vi "J1939 - Tool.vi"() -> ()   [LabVIEW 2019, in "J1939 Workspace Tool.lvlib"]
uses:
  J1939 Workspace Tool.lvlib
  NationalInstruments.VeriStand.SystemStorage
  SubModules/CAN-Streaming-Support/Source/Addon/Addon Shared/Types/Type Filter.ctl
  SubModules/CAN-Streaming-Support/Source/Addon/Addon Shared/Types/Direction Filter.ctl
  Workspace Shared/Types/UI.StateVariables.ctl
  <vilib>/NI VeriStand/Display Template Support/DisplayTemplateSupport.llb/enum_Display Template Handler Minimal To Widget Msg.ctl
  <vilib>/NI VeriStand/Execution/Workspace/SystemStateRegEventRef.ctl
  <vilib>/NI VeriStand/Execution/Workspace/Target State Info.ctl
  <vilib>/NI VeriStand/Execution/Workspace/Target State.ctl
  Workspace Shared/Types/Private Data.ctl
  <vilib>/NI/STM/TCP/TCP Connection Info.ctl
  <vilib>/NI/STM/SubVIs/MetaDataElement.ctl
  Addon/Addon Shared/Types/Error Cluster.ctl
  Addon/Addon Shared/Types/Error Types.ctl
  <vilib>/NI VeriStand/Display Template Support/DisplayTemplateSupport.llb/enum_Display Template Handler Minimal To Workspace.ctl
  <vilib>/NI VeriStand/Execution/Workspace/WorkspaceAPI.ctl
  <vilib>/NI VeriStand/Execution/Workspace/SystemStateEventRef.ctl
  Workspace Shared/Types/UI.Refs.ctl
  SubModules/CAN-Streaming-Support/Source/UIs/Workspace Shared/Types/Host Stream Queue Refs.ctl
  SubModules/CAN-Streaming-Support/Source/UIs/Workspace Shared/Types/Host Stream Queue Type.ctl
  SubModules/CAN-Streaming-Support/Source/UIs/Workspace Shared/Types/Host Stream Queue Command.ctl
  <vilib>/xnet/xnet.llb/XNET Frame CAN.ctl
  <vilib>/xnet/xnet.llb/XNET Frame Type CAN.ctl
  SubModules/CAN-Streaming-Support/Source/UIs/Workspace Shared/Types/Host Stream Engine Parameters.ctl
  SubModules/CAN-Streaming-Support/Source/Addon/Addon Shared/Types/Filter Parameters.ctl
  <vilib>/Utility/miscctls.llb/LVRowAndColumnUnsignedTypeDef.ctl
  Addon/Support Libraries/J1939 Utilities/SubVIs/Convert CAN Arb ID to J1939 ID.vi
  <vilib>/dlg_ctls.llb/Space Constant.vi
  SubModules/CAN-Streaming-Support/Source/UIs/Workspace Shared/SubVIs/Create Host Stream Refs.vi
  SubModules/CAN-Streaming-Support/Source/UIs/Workspace Shared/SubVIs/Read Host Stream.vi
  SubModules/CAN-Streaming-Support/Source/UIs/Workspace Shared/SubVIs/Cleanup Host Stream.vi
  SubModules/CAN-Streaming-Support/Source/UIs/Workspace Shared/SubVIs/Create Bus Log File.vi
  SubModules/CAN-Streaming-Support/Source/UIs/Workspace Shared/SubVIs/Write to Bus Log File.vi
  SubModules/CAN-Streaming-Support/Source/UIs/Workspace Shared/SubVIs/Convert BIN to TXT File.vi
  SubModules/CAN-Streaming-Support/Source/UIs/Workspace Shared/SubVIs/Get Next Bus Engine State.vi
  SubModules/CAN-Streaming-Support/Source/UIs/Workspace Shared/SubVIs/Get Engine Trigger State.vi
  SubModules/CAN-Streaming-Support/Source/UIs/Workspace Shared/SubVIs/Get Next Log Engine State.vi
  SubModules/CAN-Streaming-Support/Source/UIs/Workspace Shared/SubVIs/Process CAN Data.vi
  SubModules/CAN-Streaming-Support/Source/UIs/Workspace Shared/SubVIs/Process CAN State.vi
  SubModules/CAN-Streaming-Support/Source/UIs/Workspace Shared/SubVIs/Convert Frame Array to String Array.vi
  SubModules/CAN-Streaming-Support/Source/UIs/Workspace Shared/SubVIs/Convert Time to UTC String.vi
  <vilib>/Utility/error.llb/Trim Whitespace.vi
  <userlib>/_OpenG.lib/array/array.llb/Sort Array__ogtk.vi
  <userlib>/_OpenG.lib/array/array.llb/Sort 2D Array (String)__ogtk.vi
  <vilib>/Utility/libraryn.llb/Check if File or Folder Exists.vi
  <vilib>/Utility/libraryn.llb/Get File Extension.vi
  Addon/Support Libraries/J1939 Utilities/J1939 Utilities.lvlib
  Workspace Shared/J1939 Workspace Shared.lvlib
  Addon/Addon Shared/J1939 Addon Shared.lvlib
  <vilib>/NI/STM/NI STM.lvlib
  <vilib>/NI VeriStand/Execution/Workspace/NI_VS Workspace ExecutionAPI.lvlib
  SubModules/CAN-Streaming-Support/Source/Addon/Addon Shared/CAN Stream Support Shared.lvlib
  SubModules/CAN-Streaming-Support/Source/UIs/Workspace Shared/CAN Stream Support Workspace Shared.lvlib
  APIs/Host Automation API/J1939 Host Automation API.lvlib
  NationalInstruments.VeriStand.ClientAPI
panel:
  in  "NIVS.Workspace Event":refnum<event-registration>
  in  "NIVS.Gateway IP Address":string
  in  "NIVS.System Definition Root":refnum<k24>
  in  "Tab Control":T1(tab)
  in  "Refresh Continuous":bool
  in  "Clear DTC":bool
  in  "Refresh DTCs":bool
  in  "DTCs":i32(listbox)
  in  "Addresses":string(tree)
  in  "Refresh Addresses":bool
  out "Response":string
  in  "Request":bool
  in  "PGN":u32 format="%.0x"
  in  "DA":u8(ring)
  in  "Clear Array":bool
  in  "RAW":bool
  out "Priority":u8 format="%02x"
  out "SA":u8 format="%02x"
  out "PGN":u32 format="%06x"
  in  "Identifier":u32 format="%08x"
  in  "Data":u8[](array[numeric])=[0, 0, 0, 0, 0, 0, 0, 0] format="%.0x"
  in  "Host Filter":bool
  in  "Filter IDs":string caption="Filter IDs (format = x<ID>, comma separated, ID x0 = Bus Error)"
  in  "Type Filter":T2
  in  "Direction Filter":T3
  in  "Log":bool
  in  "Clear History":bool
  out "Table Control":string[][](table)
  out "Stream Connected":bool
  out "Status":string
  in  "Sort By ID":bool
  in  "Pause":bool
  in  "Enable Stream":bool
  in  "Reset Filter":bool
  out "Device":string
  in  "Errors":bool
  # "This is the root reference to the active System Definition file. You could use this to read the configuration or populate a tree with channels. You are free to close this reference, but it will be closed for you if you don't."
  # "The SystemStorageUI .NET assembly provides controls to display data configured in the System Definition file."
  # "This is the IP Address of the VeriStand Gateway to which the Workspace is connected. Use this to open all the .NET Manager references. Usually the Gateway is running on localhost, but it could be running on a neighbor's machine."
  # "This registered string User Event is used to help instruct your tool to shut down when the Workspace is closing."
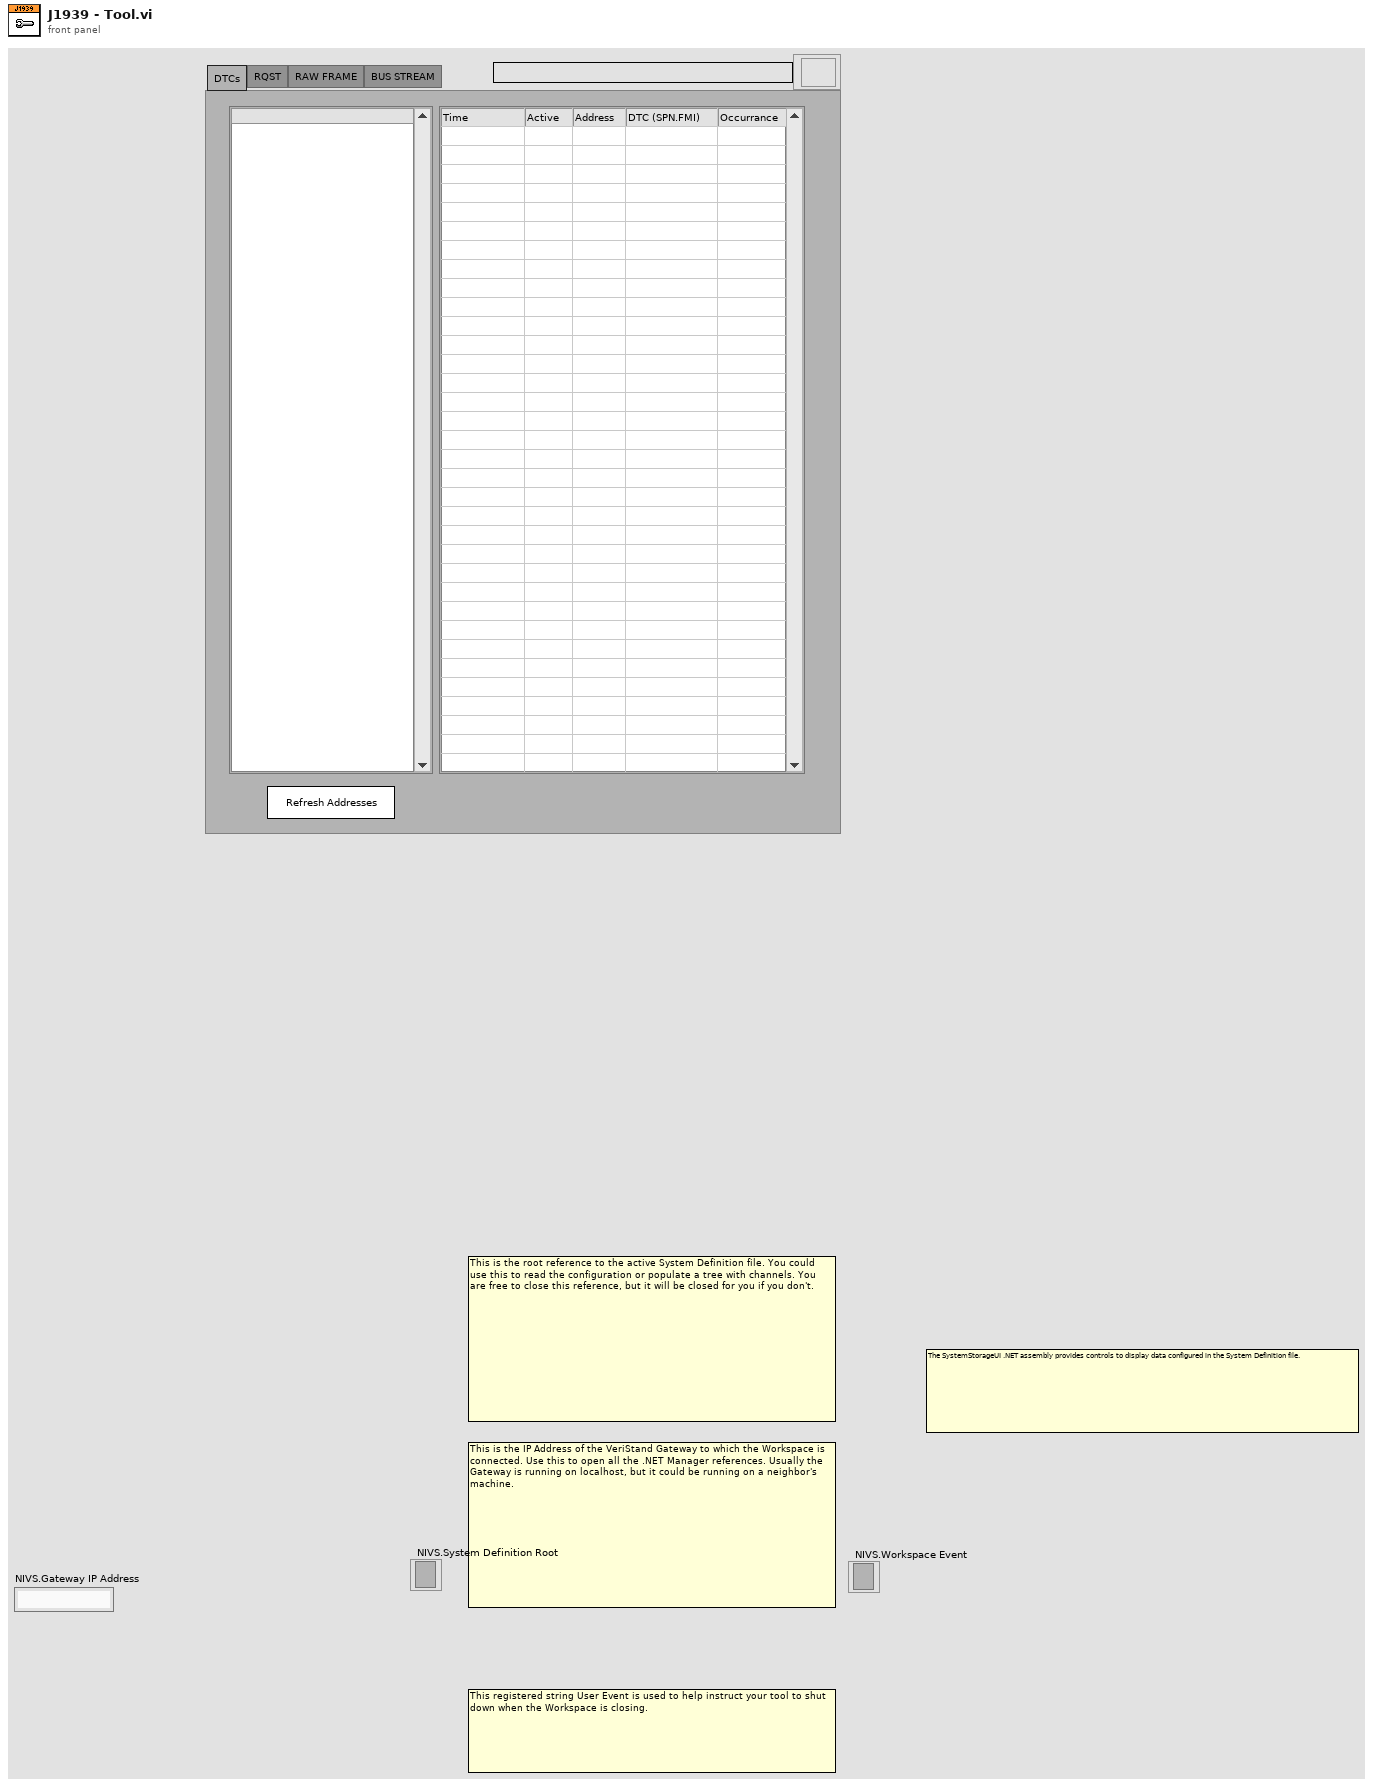
[diagram p1: front panel]
types:
  T1 = enum32{"DTCs", "RQST", "RAW FRAME", "BUS STREAM"}
  T2 = typedef "CAN Stream Support Shared.lvlib/Type Filter.ctl" = enum16{"All", "CAN Data", "CAN Remote", "CAN Bus Error", "CAN 2.0 Data", "CAN FD Data", "CAN FD+BRS Data", "J1939 Data", "Delay", "Log Trigger", "Start Trigger"}
  T3 = typedef "CAN Stream Support Shared.lvlib/Direction Filter.ctl" = enum16{"Tx/Rx", "Rx", "Tx"}
  T4 = typedef "J1939 Workspace Shared.lvlib/Private Data.ctl" = cluster{"PGN":u32, "DA":u8, "CD Path":string, "CD IP":string}
  T5 = typedef "J1939 Workspace Shared.lvlib/UI.StateVariables.ctl" = cluster{"NIVS.Gateway IP Address":string, "LaunchConfig.Ref":refnum<user-event>, "Events.Refs":cluster{"LaunchConfig":refnum<event-registration>, "SystemChange":T6, "NIVS.Workspace":refnum<event-registration>}, "State":T4, "TCP.Refs":T7, "Addresses.LUT":variant, "Errors.Q":refnum<queue>, "NIVS.SysDefRoot":refnum<k24>, "State.Notifier":refnum<user-event>, "NIVS.Workspace":T9, "DTCs.Refresh":bool, "NIVS.State.Refs":T10, "UI.Refs":T11, "Addon.Connected":bool, "DTCs.Timer":u32, "Mode.Tool?":bool, "Stream.Qs":T12, "NIVS.SysDef":path}
  T6 = typedef "NI_VS Workspace ExecutionAPI.lvlib/SystemStateRegEventRef.ctl" = refnum<event-registration>
  T7 = typedef "NI STM.lvlib/TCP Connection Info.ctl" = cluster{"connection ID":refnum<k5>, "meta data":T8[]}
  T8 = typedef "NI STM.lvlib/MetaDataElement.ctl" = string
  T9 = typedef "NI_VS Workspace ExecutionAPI.lvlib/WorkspaceAPI.ctl" = refnum<k24>
  T10 = typedef "NI_VS Workspace ExecutionAPI.lvlib/SystemStateEventRef.ctl" = cluster{"CustDatRef":refnum<user-event>, "EvtRef":refnum<k27>, "Target State User Event":refnum<user-event>}
  T11 = typedef "J1939 Workspace Shared.lvlib/UI.Refs.ctl" = cluster{"ParentVI":refnum<vi>, "DTCs":refnum<vi>, "Addresses":refnum<vi>, "Device":refnum<vi>, "Data":refnum<vi>, "Identifier":refnum<vi>, "PGN":refnum<vi>, "DA":refnum<vi>, "Refresh Continuous":refnum<vi>, "Errors":refnum<vi>, "Refresh Addresses":refnum<vi>, "Refresh DTCs":refnum<vi>, "Clear DTC":refnum<vi>, "Request":refnum<vi>, "Clear Array":refnum<vi>, "RAW":refnum<vi>, "SA":refnum<vi>, "PGN Ind":refnum<vi>, "Priority":refnum<vi>, "Response":refnum<vi>, "Reset Filter":refnum<vi>, "Enable Stream":refnum<vi>, "Log":refnum<vi>, "Clear History":refnum<vi>, "Sort By ID":refnum<vi>, "Pause":refnum<vi>, "Table Control":refnum<vi>, "Status":refnum<vi>, "Type Filter":refnum<vi>, "Filter IDs":refnum<vi>, "Host Filter":refnum<vi>, "Direction Filter":refnum<vi>, "Stream Connected":refnum<vi>}
  T12 = typedef "CAN Stream Support Workspace Shared.lvlib/Host Stream Queue Refs.ctl" = cluster{"Cmd Q":refnum<queue>, "XNET Frames":refnum<queue>}
  T13 = typedef "CAN Stream Support Workspace Shared.lvlib/Host Stream Engine Parameters.ctl" = cluster{"Host Filter":bool, "Filter Parameters":T14, "Sort By ID":bool, "Pause":bool, "Clear History":bool, "Log":bool}
  T14 = typedef "CAN Stream Support Shared.lvlib/Filter Parameters.ctl" = cluster{"ID Filters":u32[], "Direction Filter":T3, "Type Filter":T2}
  T15 = typedef "CAN Stream Support Workspace Shared.lvlib/Host Stream Data.ctl" = cluster{"Connected":bool, "Bus Data Update":bool, "Bus Data":string[][], "Bus Status":string, "Bus Warning":bool, "Log Status":string}
  T16 = enum8{"Enabled", "Disabled", "Disabled and Grayed Out"}
  T17 = typedef "enum_Display Template Handler Minimal To Workspace.ctl" = cluster{"Operation":enum16{"SetCustomData", "DeleteItem"}, "Data":variant}
  T18 = typedef "LVRowAndColumnUnsignedTypeDef.ctl" = cluster{"Row":u32, "Column":u32}
  T19 = cluster{"LaunchConfig":refnum<event-registration>, "SystemChange":T6, "NIVS.Workspace":refnum<event-registration>}
  T20 = typedef "enum_Display Template Handler Minimal To Widget Msg.ctl" = enum16{"Stop", "LaunchConfigDialog"}
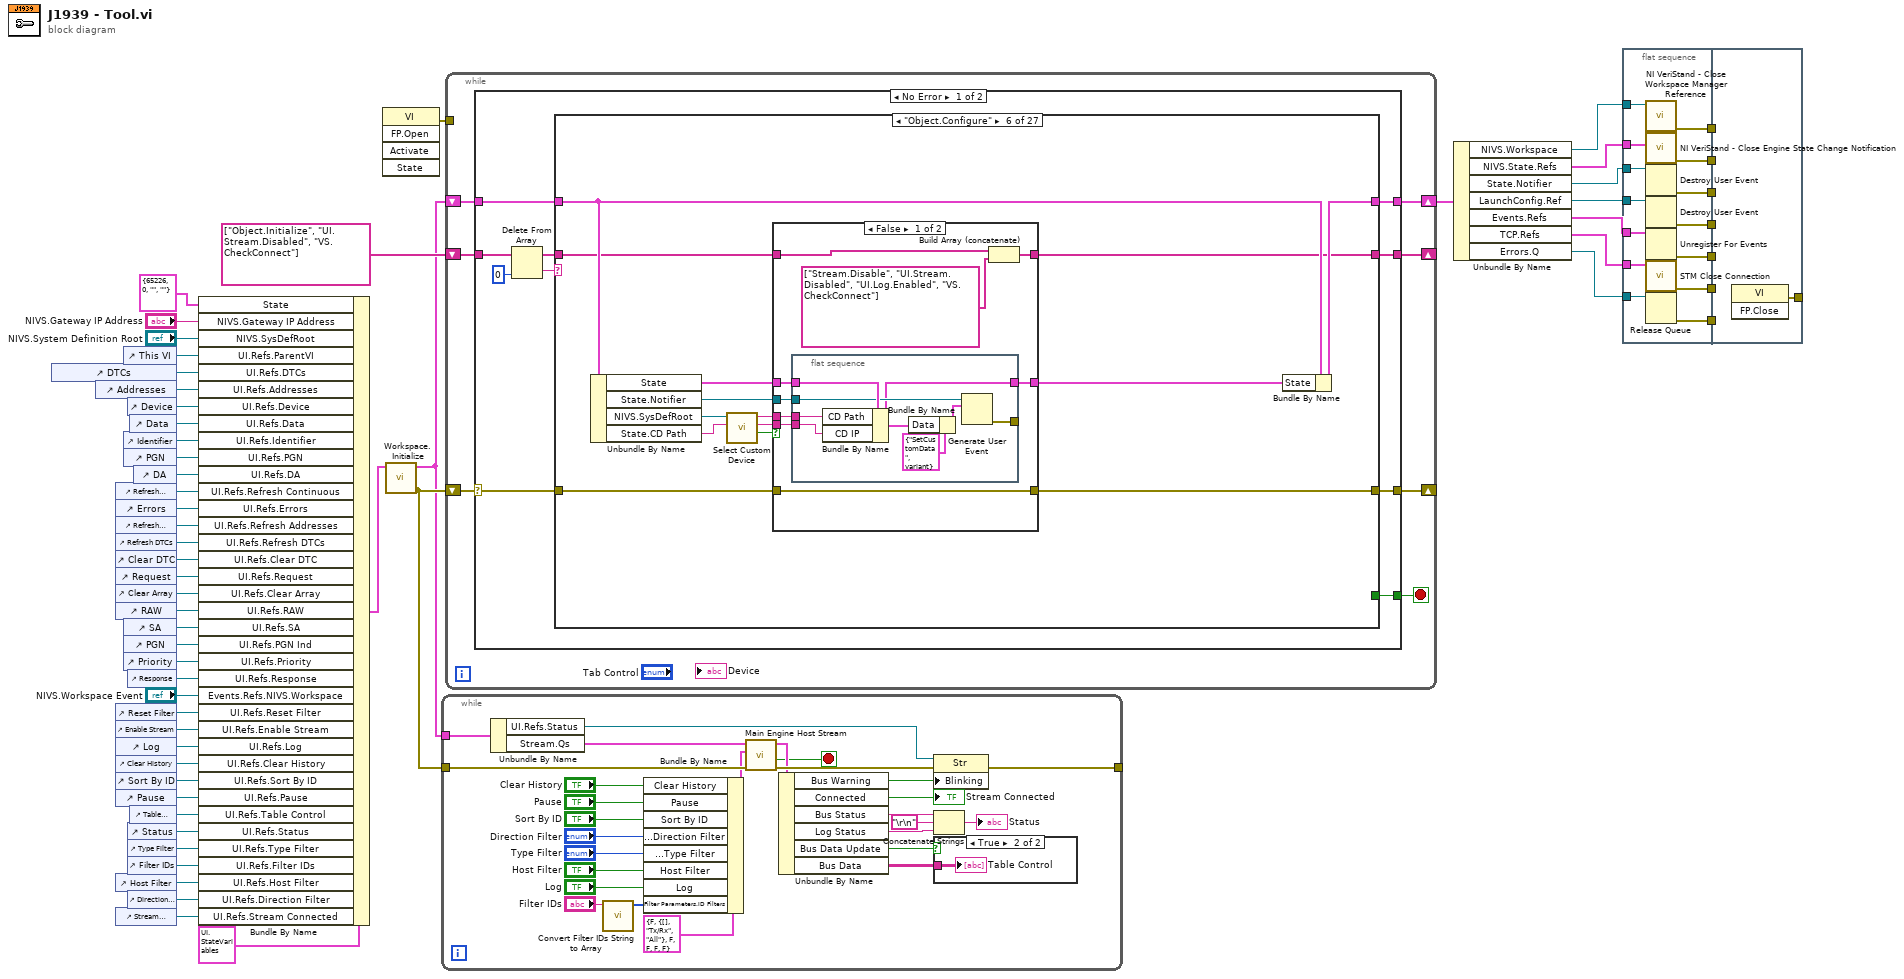
[diagram p0: block diagram]
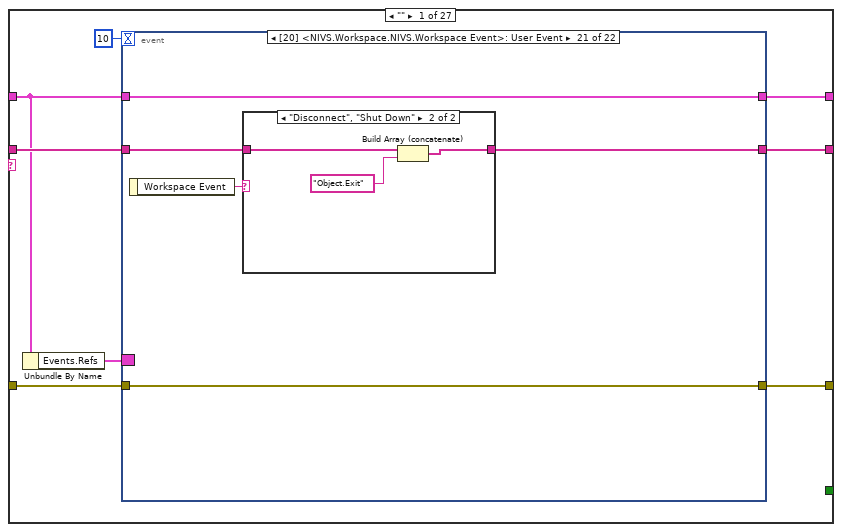
[diagram p3: hidden frame]
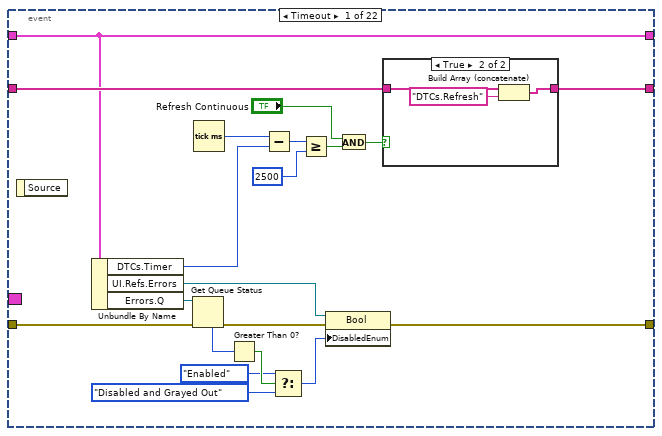
[diagram p4: hidden frame]
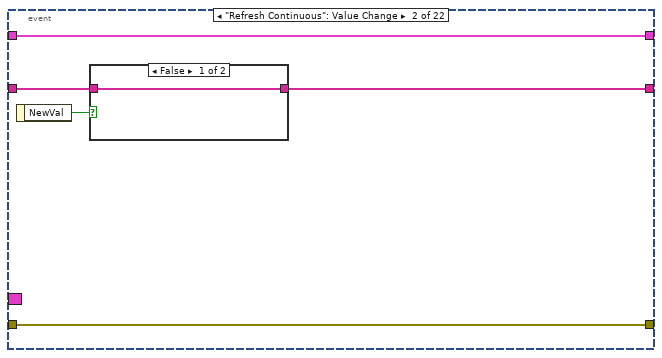
[diagram p6: hidden frame]
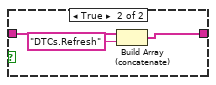
[diagram p7: hidden frame]
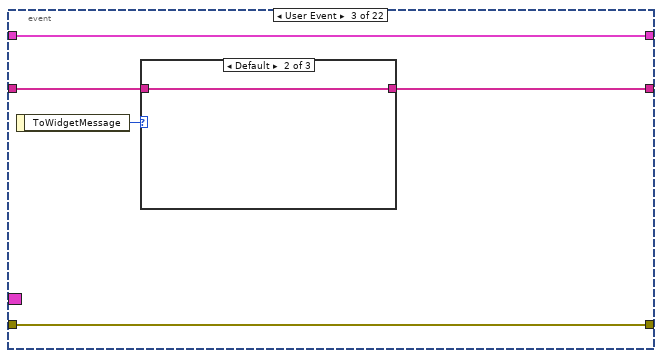
[diagram p8: hidden frame]
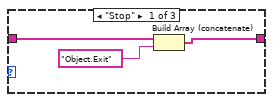
[diagram p9: hidden frame]
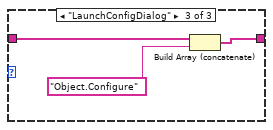
[diagram p10: hidden frame]
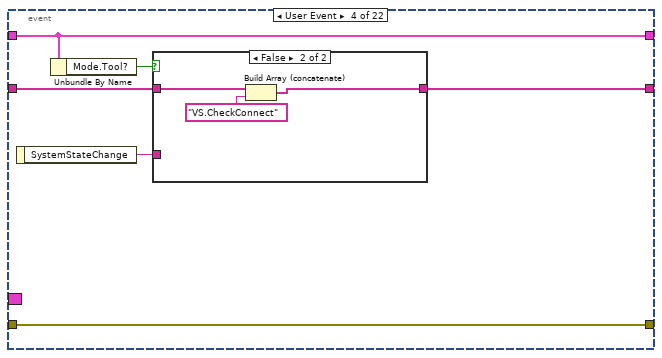
[diagram p11: hidden frame]
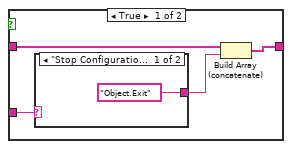
[diagram p12: hidden frame]
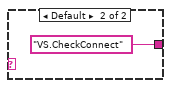
[diagram p13: hidden frame]
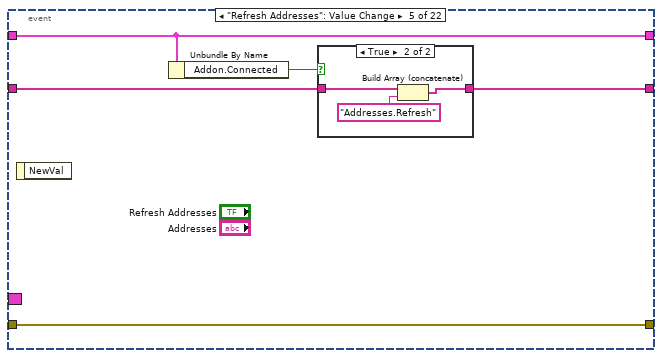
[diagram p14: hidden frame]
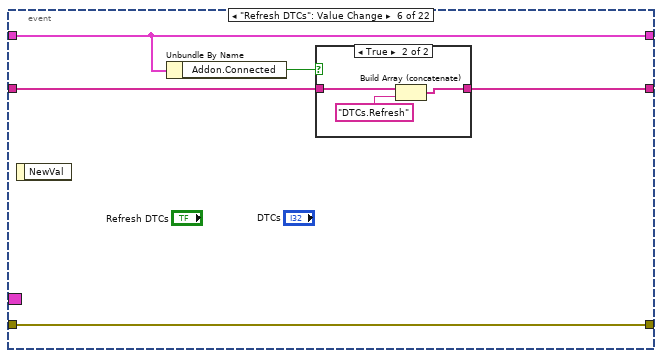
[diagram p16: hidden frame]
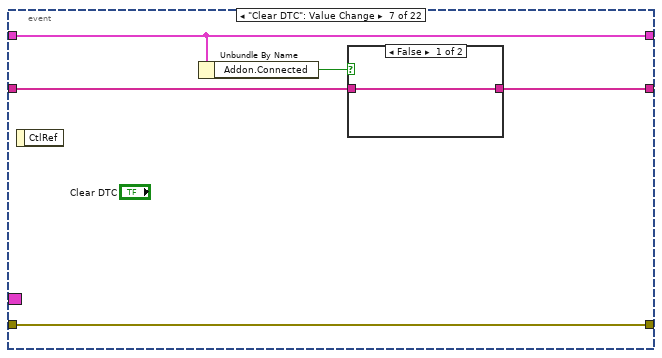
[diagram p18: hidden frame]
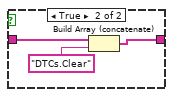
[diagram p19: hidden frame]
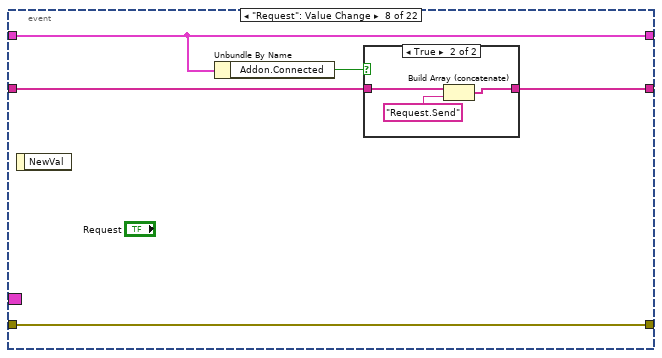
[diagram p20: hidden frame]
diagram:
  n1 = control-ref of="DTCs"() -> (w53:refnum<vi>)
  n2 = control-ref of="Addresses"() -> (w52:refnum<vi>)
  n3 = control-ref of="Refresh Continuous"() -> (w46:refnum<vi>)
  n4 = control-ref of="Errors"() -> (w45:refnum<vi>)
  n5 = control-ref of="Refresh Addresses"() -> (w44:refnum<vi>)
  n6 = control-ref of="Refresh DTCs"() -> (w43:refnum<vi>)
  n7 = control-ref of="Clear DTC"() -> (w42:refnum<vi>)
  n8 = control-ref of="Request"() -> (w41:refnum<vi>)
  n9 = control-ref of="Clear Array"() -> (w40:refnum<vi>)
  n10 = control-ref of="RAW"() -> (w39:refnum<vi>)
  n11 = control-ref of="Reset Filter"() -> (w15:refnum<vi>)
  n12 = control-ref of="Enable Stream"() -> (w14:refnum<vi>)
  n13 = control-ref of="Log"() -> (w13:refnum<vi>)
  n14 = control-ref of="Clear History"() -> (w12:refnum<vi>)
  n15 = control-ref of="Sort By ID"() -> (w11:refnum<vi>)
  n16 = control-ref of="Pause"() -> (w10:refnum<vi>)
  n17 = control-ref of="Host Filter"() -> (w5:refnum<vi>)
  n18 = control-ref of="Stream Connected"() -> (w3:refnum<vi>)
  n19 = control-ref of="This VI"() -> (w54:refnum<vi>)
  n20 = control-ref of="Identifier"() -> (w49:refnum<vi>)
  n21 = control-ref of="PGN"() -> (w48:refnum<vi>)
  n22 = control-ref of="SA"() -> (w19:refnum<vi>)
  n23 = control-ref of="PGN"() -> (w18:refnum<vi>)
  n24 = control-ref of="Priority"() -> (w17:refnum<vi>)
  n25 = control-ref of="Device"() -> (w51:refnum<vi>)
  n26 = control-ref of="Response"() -> (w16:refnum<vi>)
  n27 = control-ref of="Status"() -> (w8:refnum<vi>)
  n28 = control-ref of="Type Filter"() -> (w7:refnum<vi>)
  n29 = control-ref of="Filter IDs"() -> (w6:refnum<vi>)
  n30 = control-ref of="Direction Filter"() -> (w4:refnum<vi>)
  n31 = control-ref of="Data"() -> (w50:refnum<vi>)
  n32 = control-ref of="Table Control"() -> (w9:refnum<vi>)
  n33 = control-ref of="DA"() -> (w47:refnum<vi>)
  n34 = Bundle By Name(cluster=T5 {"NIVS.Gateway IP Address"="", "LaunchConfig.Ref"=refnum, "Events.Refs"={"LaunchConfig"=refnum, "SystemChange"=refnum, "NIVS.Workspace"=refnum}, "State"={"PGN"=0, "DA"=0, "CD Path"="", "CD IP"=""}, "TCP.Refs"={"connection ID"=refnum, "meta data"=[]}, "Addresses.LUT"=variant, "Errors.Q"=refnum, "NIVS.SysDefRoot"=refnum, "State.Notifier"=refnum, "NIVS.Workspace"=refnum, "DTCs.Refresh"=FALSE, "NIVS.State.Refs"={"CustDatRef"=refnum, "EvtRef"=refnum, "Target State User Event"=refnum}, "UI.Refs"={"ParentVI"=refnum, "DTCs"=refnum, "Addresses"=refnum, "Device"=refnum, "Data"=refnum, "Identifier"=refnum, "PGN"=refnum, "DA"=refnum, "Refresh Continuous"=refnum, "Errors"=refnum, "Refresh Addresses"=refnum, "Refresh DTCs"=refnum, "Clear DTC"=refnum, "Request"=refnum, "Clear Array"=refnum, "RAW"=refnum, "SA"=refnum, "PGN Ind"=refnum, "Priority"=refnum, "Response"=refnum, "Reset Filter"=refnum, "Enable Stream"=refnum, "Log"=refnum, "Clear History"=refnum, "Sort By ID"=refnum, "Pause"=refnum, "Table Control"=refnum, "Status"=refnum, "Type Filter"=refnum, "Filter IDs"=refnum, "Host Filter"=refnum, "Direction Filter"=refnum, "Stream Connected"=refnum}, "Addon.Connected"=FALSE, "DTCs.Timer"=0, "Mode.Tool?"=FALSE, "Stream.Qs"={"Cmd Q"=refnum, "XNET Frames"=refnum}, "NIVS.SysDef"=path ""}, "State"=T4 {"PGN"=65226, "DA"=0, "CD Path"="", "CD IP"=""} ("Cluster"), "NIVS.Gateway IP Address"="NIVS.Gateway IP Address", "NIVS.SysDefRoot"="NIVS.System Definition Root", "UI.Refs.ParentVI"=w54, "UI.Refs.DTCs"=w53, "UI.Refs.Addresses"=w52, "UI.Refs.Device"=w51, "UI.Refs.Data"=w50, "UI.Refs.Identifier"=w49, "UI.Refs.PGN"=w48, "UI.Refs.DA"=w47, "UI.Refs.Refresh Continuous"=w46, "UI.Refs.Errors"=w45, "UI.Refs.Refresh Addresses"=w44, "UI.Refs.Refresh DTCs"=w43, "UI.Refs.Clear DTC"=w42, "UI.Refs.Request"=w41, "UI.Refs.Clear Array"=w40, "UI.Refs.RAW"=w39, "UI.Refs.SA"=w19, "UI.Refs.PGN Ind"=w18, "UI.Refs.Priority"=w17, "UI.Refs.Response"=w16, "Events.Refs.NIVS.Workspace"="NIVS.Workspace Event", "UI.Refs.Reset Filter"=w15, "UI.Refs.Enable Stream"=w14, "UI.Refs.Log"=w13, "UI.Refs.Clear History"=w12, "UI.Refs.Sort By ID"=w11, "UI.Refs.Pause"=w10, "UI.Refs.Table Control"=w9, "UI.Refs.Status"=w8, "UI.Refs.Type Filter"=w7, "UI.Refs.Filter IDs"=w6, "UI.Refs.Host Filter"=w5, "UI.Refs.Direction Filter"=w4, "UI.Refs.Stream Connected"=w3) -> (w55:T5)
  n35 = invoke class="VI" method="FP.Open"() -> (error out=w27:errorcluster)  [unwired: 5 in, 4 out]
  n36 = call "Workspace.Initialize.vi"("State"=w55) -> ("error out"=w2:errorcluster, "State"=w1:T5)  [unwired: 9 in]
  n37 = while {
    tunnel: w2 -> [w64]
    tunnel: w1 -> [w85]
    tunnel: [w81] -> _
    stop <- w61 stop-if-true
    n38 = Unbundle By Name(w85) -> ("UI.Refs.Status"=w84:refnum<vi>, "Stream.Qs"=w59:T12)
    n39 = call "Convert Filter IDs String to Array.vi"("Filter IDs"="Filter IDs") -> ("Filter IDs"=w65:u32[])  [unwired: 10 in]
    n40 = Bundle By Name(cluster=T13 {"Host Filter"=FALSE, "Filter Parameters"={"ID Filters"=[], "Direction Filter"=enum."Tx/Rx", "Type Filter"=enum."All"}, "Sort By ID"=FALSE, "Pause"=FALSE, "Clear History"=FALSE, "Log"=FALSE} ("Host Parameters"), "Clear History"="Clear History", "Pause"="Pause", "Sort By ID"="Sort By ID", "Filter Parameters.Direction Filter"="Direction Filter", "Filter Parameters.Type Filter"="Type Filter", "Host Filter"="Host Filter", "Log"="Log", "Filter Parameters.ID Filters"=w65) -> (w60:T13)
    n41 = call "Main Engine Host Stream.vi"("error in (no error)"=w64, "Host Parameters"=w60, "Q Refs"=w59) -> ("error out"=w63:errorcluster, "Exit"=w61:bool, "Stream"=w62:T15)  [unwired: 6 in]
    n42 = Unbundle By Name(w62) -> ("Bus Warning"=w83:bool, "Connected"=→"Stream Connected":bool, "Bus Status"=w76:string, "Log Status"=w72:string, "Bus Data Update"=w71:bool, "Bus Data"=w70:string[][])
    n43 = property class="Str"(reference=w84, error in=w63, "Blinking"=w83) -> (error out=w81:errorcluster)  [unwired: 1 out]
    n44 = Concatenate Strings(w76, "\r\n", w72) -> (→"Status":string)
    n45 = case shown="True" w71 {
      tunnel: w70 -> [_ w86]
      frame False {
      }
      frame True {
        "Table Control" <- w86
      }
    }
  }
  n46 = while {
    shift-right: [w91] -> _
    shift-left: w2 -> [w92]
    shift-right: [w87] -> w37
    shift-left: w1 -> [w90]
    shift-right: [w88] -> _
    shift-left: string[] ["Object.Initialize", "UI.Stream.Disabled", "VS.CheckConnect"] -> [w89]
    tunnel: w27 -> [_]
    stop <- w93 stop-if-true
    n47 = case shown="No Error" w92 {
      selector: w92 -> [w94 w684]
      tunnel: [w103 FALSE] -> w93
      tunnel: [w95 w682] -> w91
      tunnel: w90 -> [w102 w679]
      tunnel: w89 -> [w100 w680]
      tunnel: [w97 w680] -> w88
      tunnel: [w96 w679] -> w87
      frame No Error {
        n48 = Delete From Array(array=w100, index=0) -> (deleted portion=w99:string, array with subset deleted=w98:string[])  [unwired: 1 in]
        n49 = case shown="\"Object.Configure\"" w99 {
          selector: w99 -> [_ _ _ _ _ _ _ _ _ _ _ _ _ _ _ _ _ _ _ _ _ _ _ _ _ _ w674]
          tunnel: [_ _ _ _ _ _ _ _ TRUE _ _ _ _ _ _ _ _ _ _ _ _ _ _ _ _ _ _] -> w103
          tunnel: w102 -> [w105 w338 w347 w364 w393 w398 w432 w460 w462 w471 w494 w510 w517 w533 w544 w562 w569 w578 w586 w598 w608 w618 w622 w643 w648 w665 w677]
          tunnel: w98 -> [w109 w345 w357 w373 w394 w396 w438 w456 w466 w469 w497 w514 w526 w543 w559 w565 w570 w579 w587 w594 w615 w619 w621 w646 w659 w672 w678]
          tunnel: [w110 w345 w357 w373 w394 w395 w437 w456 w466 w468 w497 w514 w526 w543 w559 w565 w570 w579 w587 w594 w615 w619 w621 w646 w659 w672 w678] -> w97
          tunnel: [w108 w335 w346 w374 w393 w397 w431 w459 w462 w472 w494 w510 w517 w533 w544 w562 w569 w578 w585 w595 w609 w618 w622 w643 w648 w666 w677] -> w96
          tunnel: [w107 w334 w356 w359 w392 w401 w434 w455 w464 w480 w496 w513 w525 w542 w558 w561 w567 w574 w580 w593 w610 w617 w620 w645 w647 w667 w676] -> w95
          tunnel: w94 -> [w106 w334 w356 w360 w391 w402 w433 w455 w463 w481 w495 w513 w525 w542 w558 w560 w566 w573 w580 w593 w611 w616 w623 w644 w649 w668 w676]
          frame "" {
            n50 = Unbundle By Name(w105) -> ("Events.Refs"=w104:T19)
            n51 = event shown="[20] <NIVS.Workspace.NIVS.Workspace Event>: User Event" {
              selector: w104 -> [_ _ _ _ _ _ _ _ _ _ _ _ _ _ _ _ _ _ _ _ _ _]
              dyn-events: _ -> [_ _ _ _ _ _ _ _ _ _ _ _ _ _ _ _ _ _ _ _ _ _]
              timeout: 10 -> [_ _ _ _ _ _ _ _ _ _ _ _ _ _ _ _ _ _ _ _ _ _]
              tunnel: w105 -> [w120 w139 w149 w158 w175 w183 w190 w201 w210 w219 w228 w232 w239 w249 w251 w266 w278 w287 w295 w310 w324 w333]
              tunnel: [w121 w137 w145 w161 w173 w181 w191 w199 w208 w217 w227 w233 w241 w245 w254 w264 w277 w286 w298 w308 w321 w330] -> w110
              tunnel: w109 -> [w122 w138 w146 w162 w174 w182 w192 w200 w209 w218 w230 w233 w241 w246 w253 w263 w276 w285 w297 w309 w322 w331]
              tunnel: [w120 w139 w149 w158 w175 w183 w190 w201 w210 w219 w228 w232 w239 w249 w251 w266 w278 w287 w295 w310 w324 w333] -> w108
              tunnel: [w114 w140 w148 w159 w176 w185 w194 w203 w212 w221 w229 w231 w240 w248 w255 w269 w280 w289 w299 w312 w323 w332] -> w107
              tunnel: w106 -> [w116 w140 w148 w159 w176 w185 w194 w203 w212 w221 w229 w231 w240 w248 w255 w269 w280 w289 w299 w312 w323 w332]
              event Timeout {
                n52 = event-data() -> ()  [unwired: 2 out]
                n53 = Unbundle By Name(w120) -> ("DTCs.Timer"=w113:u32, "UI.Refs.Errors"=w118:refnum<vi>, "Errors.Q"=w119:refnum<queue>)
                n54 = Get Queue Status(queue=w119, error in (no error)=w116) -> (error out=w117:errorcluster, # elements in queue=w131:i32)  [unwired: 1 in, 6 out]
                n55 = Tick Count (ms)() -> (millisecond timer value=w125:u32)
                n56 = Greater Than 0?(x=w131) -> (x > 0?=w130:bool)
                n57 = Subtract(x=w125, y=w113) -> (x-y=w127:u32)
                n58 = Select(t=T16."Enabled" ("Disabled"), s=w130, f=T16."Disabled and Grayed Out") -> (s? t:f=w115:T16)
                n59 = Greater Or Equal?(x=w127, y=u32 2500) -> (x >= y?=w112:bool)
                n60 = property class="Bool"(reference=w118, error in=w117, "DisabledEnum"=w115) -> (error out=w114:errorcluster)  [unwired: 1 out]
                n61 = And(x="Refresh Continuous", y=w112) -> (x .and. y?=w123:bool)
                n62 = case shown="True" w123 {
                  tunnel: w122 -> [w132 w134]
                  tunnel: [w132 w133] -> w121
                  frame False {
                  }
                  frame True {
                    n63 = Build Array (concatenate)(w134, "DTCs.Refresh" ("NewVal")) -> (w133:string[])
                  }
                }
              }
              event "Refresh Continuous": Value Change {
                n64 = event-data() -> ("NewVal"=w136:bool)  [unwired: 1 out]
                n65 = case shown="False" w136 {
                  tunnel: w138 -> [w141 w143]
                  tunnel: [w141 w142] -> w137
                  frame False {
                  }
                  frame True {
                    n66 = Build Array (concatenate)(w143, "DTCs.Refresh" ("NewVal")) -> (w142:string[])
                  }
                }
              }
              event User Event {
                n67 = event-data() -> ("ToWidgetMessage"=w147:T20)  [unwired: 1 out]
                n68 = case shown="Default" w147 {
                  tunnel: w146 -> [w152 w153 w156]
                  tunnel: [w151 w153 w155] -> w145
                  frame "Stop" {
                    n69 = Build Array (concatenate)(w152, "Object.Exit") -> (w151:string[])
                  }
                  frame Default {
                  }
                  frame "LaunchConfigDialog" {
                    n70 = Build Array (concatenate)(w156, "Object.Configure") -> (w155:string[])
                  }
                }
              }
              event User Event {
                n71 = event-data() -> ("SystemStateChange"=w157:string)  [unwired: 1 out]
                n72 = Unbundle By Name(w158) -> ("Mode.Tool?"=w160:bool)
                n73 = case shown="False" w160 {
                  tunnel: w162 -> [w166 w171]
                  tunnel: [w165 w170] -> w161
                  tunnel: w157 -> [w164 _]
                  frame True {
                    # "System state not connected"
                    n74 = case shown="\"Stop Configuration\"" w164 {
                      tunnel: ["Object.Exit" "VS.CheckConnect"] -> w163
                      frame "Stop Configuration" {
                      }
                      frame Default {
                      }
                    }
                    n75 = Build Array (concatenate)(w166, w163) -> (w165:string[])
                  }
                  frame False {
                    # "System state is connected"
                    n76 = Build Array (concatenate)(w171, "VS.CheckConnect") -> (w170:string[])
                  }
                }
              }
              event "Refresh Addresses": Value Change {
                n77 = event-data() -> ()  [unwired: 2 out]
                n78 = Unbundle By Name(w175) -> ("Addon.Connected"=w172:bool)
                n79 = case shown="True" w172 {
                  tunnel: w174 -> [w177 w179]
                  tunnel: [w177 w178] -> w173
                  frame False {
                  }
                  frame True {
                    n80 = Build Array (concatenate)(w179, "Addresses.Refresh") -> (w178:string[])
                  }
                }
              }
              event "Refresh DTCs": Value Change {
                n81 = event-data() -> ()  [unwired: 2 out]
                n82 = Unbundle By Name(w183) -> ("Addon.Connected"=w184:bool)
                n83 = case shown="True" w184 {
                  tunnel: w182 -> [w186 w188]
                  tunnel: [w186 w187] -> w181
                  frame False {
                  }
                  frame True {
                    n84 = Build Array (concatenate)(w188, "DTCs.Refresh") -> (w187:string[])
                  }
                }
              }
              event "Clear DTC": Value Change {
                n85 = event-data() -> ()  [unwired: 2 out]
                n86 = Unbundle By Name(w190) -> ("Addon.Connected"=w193:bool)
                n87 = case shown="False" w193 {
                  tunnel: w192 -> [w195 w197]
                  tunnel: [w195 w196] -> w191
                  frame False {
                  }
                  frame True {
                    n88 = Build Array (concatenate)(w197, "DTCs.Clear") -> (w196:string[])
                  }
                }
              }
              event "Request": Value Change {
                n89 = event-data() -> ()  [unwired: 2 out]
                n90 = Unbundle By Name(w201) -> ("Addon.Connected"=w202:bool)
                n91 = case shown="True" w202 {
                  tunnel: w200 -> [w204 w206]
                  tunnel: [w204 w205] -> w199
                  frame False {
                  }
                  frame True {
                    n92 = Build Array (concatenate)(w206, "Request.Send") -> (w205:string[])
                  }
                }
              }
              event "RAW": Value Change {
                n93 = event-data() -> ()  [unwired: 2 out]
                n94 = Unbundle By Name(w210) -> ("Addon.Connected"=w211:bool)
                n95 = case shown="True" w211 {
                  tunnel: w209 -> [w213 w215]
                  tunnel: [w213 w214] -> w208
                  frame False {
                  }
                  frame True {
                    n96 = Build Array (concatenate)(w215, "Raw.Send") -> (w214:string[])
                  }
                }
              }
              event "Clear Array": Value Change {
                n97 = event-data() -> ()  [unwired: 2 out]
                n98 = Unbundle By Name(w219) -> ("Addon.Connected"=w220:bool)
                n99 = case shown="True" w220 {
                  tunnel: w218 -> [w222 w224]
                  tunnel: [w222 w223] -> w217
                  frame False {
                  }
                  frame True {
                    n100 = Build Array (concatenate)(w224, "Raw.Clear") -> (w223:string[])
                  }
                }
              }
              event "Addresses": Value Change {
                n101 = event-data() -> ()  [unwired: 2 out]
                n102 = Build Array (concatenate)(w230, "DTCs.Refresh" ("NewVal")) -> (w227:string[])
              }
              event "Identifier": Value Change {
                n103 = event-data() -> ("NewVal"=w234:u32)  [unwired: 1 out]
                n104 = call-poly "Common Conversions.vi"("Arb ID"=w234) -> ("Priority"=→"Priority":u8, "PGN"=→"PGN":u32, "Source Address"=→"SA":u8)  [unwired: 11 in, 1 out]
              }
              event "Errors": Value Change {
                n105 = event-data() -> ()  [unwired: 2 out]
                n106 = Unbundle By Name(w239) -> ("Errors.Q"=w238:refnum<queue>)
                n107 = flat-sequence {
                  tunnel: [w243] -> w242
                  tunnel: w238 -> [w243]
                  frame #0 {
                  }
                }
                n108 = call "Error Display.vi"("queue out"=w242) -> ()  [unwired: 11 in]
              }
              event Panel Close? {
                n109 = event-data() -> ()  [unwired: 5 out]
                n110 = Build Array (concatenate)(w246, "Object.Exit") -> (w245:string[])
                n111 = event-data("Discard?"=TRUE) -> ()  [unwired: 1 in, 1 out]
              }
              event "Enable Stream": Value Change {
                n112 = event-data() -> ()  [unwired: 2 out]
                n113 = Unbundle By Name(w251) -> ("Addon.Connected"=w250:bool)
                n114 = case shown="True" w250 {
                  tunnel: w253 -> [w256 w259]
                  tunnel: [w256 w258] -> w254
                  tunnel: "Enable Stream" -> [_ w257]
                  frame False {
                  }
                  frame True {
                    n115 = case shown="True" w257 {
                      tunnel: [string[] ["Stream.Enable", "UI.Stream.Enabled"] string[] ["Stream.Disable", "UI.Stream.Disabled"]] -> w260
                      frame True {
                      }
                      frame False {
                      }
                    }
                    n116 = Build Array (concatenate)(w259, w260) -> (w258:string[])
                  }
                }
              }
              event "Filter IDs": Value Change {
                n117 = event-data() -> ()  [unwired: 2 out]
                n118 = Unbundle By Name(w266) -> ("Addon.Connected"=w268:bool)
                n119 = local read "Host Filter"() -> (w265:bool)
                n120 = Compound Arithmetic op=AND(invert w265, w268) -> (w267:bool)
                n121 = case shown="True" w267 {
                  tunnel: w263 -> [w270 w274]
                  tunnel: [w271 w273] -> w264
                  frame False {
                    n122 = Build Array (concatenate)(w270, "Stream.Table.GoUp") -> (w271:string[])
                  }
                  frame True {
                    n123 = Build Array (concatenate)(w274, string[] ["Stream.Filter.Send", "Stream.Table.GoUp"]) -> (w273:string[])
                  }
                }
              }
              event "Clear History", "Sort By ID": Value Change {
                n124 = event-data() -> ()  [unwired: 2 out]
                n125 = Unbundle By Name(w278) -> ("Addon.Connected"=w279:bool)
                n126 = case shown="True" w279 {
                  tunnel: [w281 w284] -> w277
                  tunnel: w276 -> [w281 w283]
                  frame False {
                  }
                  frame True {
                    n127 = Build Array (concatenate)(w283, "Stream.Table.GoUp") -> (w284:string[])
                  }
                }
              }
              event "Reset Filter": Value Change {
                n128 = event-data() -> ()  [unwired: 2 out]
                n129 = Unbundle By Name(w287) -> ("Addon.Connected"=w288:bool)
                n130 = case shown="True" w288 {
                  tunnel: w285 -> [w290 w292]
                  tunnel: [w290 w291] -> w286
                  frame False {
                  }
                  frame True {
                    n131 = Build Array (concatenate)(w292, string[] ["Stream.Filter.Reset", "Stream.Table.GoUp"]) -> (w291:string[])
                  }
                }
              }
              event "Host Filter": Value Change {
                n132 = event-data() -> ("NewVal"=w296:bool)  [unwired: 1 out]
                n133 = Unbundle By Name(w295) -> ("Addon.Connected"=w294:bool)
                n134 = case shown="True" w294 {
                  tunnel: w297 -> [w300 w303]
                  tunnel: [w300 w302] -> w298
                  tunnel: w296 -> [_ w301]
                  frame False {
                  }
                  frame True {
                    n135 = case shown="False" w301 {
                      tunnel: [string[] ["Stream.Filter.Send", "Stream.Table.GoUp"] string[] ["Stream.Filter.Clear", "Stream.Table.GoUp"]] -> w304
                      frame False {
                      }
                      frame True {
                      }
                    }
                    n136 = Build Array (concatenate)(w303, w304) -> (w302:string[])
                  }
                }
              }
              event "Log": Value Change {
                n137 = event-data() -> ("NewVal"=w307:bool)  [unwired: 1 out]
                n138 = Unbundle By Name(w310) -> ("Addon.Connected"=w311:bool)
                n139 = case shown="True" w311 {
                  tunnel: w309 -> [w313 w316]
                  tunnel: [w313 w315] -> w308
                  tunnel: w307 -> [_ w314]
                  frame False {
                  }
                  frame True {
                    n140 = case shown="False" w314 {
                      tunnel: [string[] ["UI.Log.Disabled"] string[] ["UI.Log.Enabled"]] -> w317
                      frame False {
                      }
                      frame True {
                      }
                    }
                    n141 = Build Array (concatenate)(w316, w317) -> (w315:string[])
                  }
                }
              }
              event User Event {
                n142 = event-data() -> ("Workspace Event"=w320:string)  [unwired: 1 out]
                n143 = case shown="\"Disconnect\", \"Shut Down\"" w320 {
                  tunnel: w322 -> [w325 w328]
                  tunnel: [w325 w327] -> w321
                  frame Default {
                  }
                  frame "Disconnect", "Shut Down" {
                    n144 = Build Array (concatenate)(w328, "Object.Exit") -> (w327:string[])
                  }
                }
              }
              event Menu Selection (User) {
                n145 = event-data() -> ("ItemTag"=w329:string)  [unwired: 1 out]
                n146 = Build Array (concatenate)(w331, w329) -> (w330:string[])
              }
            }
          }
          frame "Addresses.Refresh" {
            n147 = Unbundle By Name(w338) -> ("UI.Refs.Addresses"=w344:refnum<vi>, "UI.Refs.DA"=w343:refnum<vi>, "TCP.Refs"=w342:T7, "State"=w341:T4, "Errors.Q"=w340:refnum<queue>, "UI.Refs.ParentVI"=w339:refnum<vi>)
            n148 = call "Request Addresses Event.vi"("connection info"=w342, "DA"=w343, "Addresses"=w344, "State Variables"=w341, "Error Q"=w340, "VI Ref"=w339) -> ("connection info"=w337:T7, "Address Lookup Table Out"=w336:variant)  [unwired: 8 in]
            n149 = Bundle By Name(cluster=w338, "TCP.Refs"=w337, "Addresses.LUT"=w336) -> (w335:T5)
          }
          frame "DTCs.Clear" {
            n150 = Unbundle By Name(w347) -> ("UI.Refs.Addresses"=w350:refnum<vi>, "TCP.Refs"=w355:T7, "State"=w354:T4, "Addresses.LUT"=w353:variant, "Errors.Q"=w352:refnum<queue>, "UI.Refs.ParentVI"=w351:refnum<vi>)
            n151 = call "Clear DTCs Event.vi"("connection info"=w355, "Addresses"=w350, "State Variables"=w354, "Address Lookup Table"=w353, "Error Q"=w352, "VI Ref"=w351) -> ("connection info"=w349:T7, "Address Lookup Table Out"=w348:variant)  [unwired: 8 in]
            n152 = Bundle By Name(cluster=w347, "TCP.Refs"=w349, "Addresses.LUT"=w348) -> (w346:T5)
          }
          frame "DTCs.Refresh" {
            n153 = Unbundle By Name(w364) -> ("UI.Refs.DTCs"=w371:refnum<vi>, "UI.Refs.Addresses"=w370:refnum<vi>, "TCP.Refs"=w369:T7, "State"=w368:T4, "Addresses.LUT"=w367:variant, "Errors.Q"=w366:refnum<queue>, "UI.Refs.ParentVI"=w365:refnum<vi>, "UI.Refs.Refresh Continuous"=w361:refnum<vi>)
            n154 = property class="Bool (strict)"(reference=w361, error in=w360) -> (error out=w359:errorcluster, "Value"=w358:bool)  [unwired: 1 out]
            n155 = Not(x=w358) -> (.not. x?=w372:bool)
            n156 = flat-sequence {
              tunnel: w367 -> [w387]
              tunnel: w369 -> [w385]
              tunnel: w368 -> [w383]
              tunnel: w372 -> [w382]
              tunnel: [w386] -> w377
              tunnel: [w384] -> w376
              tunnel: w371 -> [w381]
              tunnel: w370 -> [w380]
              tunnel: w366 -> [w379]
              tunnel: w365 -> [w378]
              tunnel: [w389] -> w362
              tunnel: [w390] -> w363
              tunnel: w377 -> [w390]
              tunnel: w376 -> [w389]
              tunnel: [w388] -> w375
              frame #0 {
                n157 = call "Refresh DTCs Event.vi"("connection info"=w385, "Addresses"=w380, "DTCs"=w381, "State Variables"=w383, "Address Lookup Table"=w387, "To Top (T)"=w382, "Error Q"=w379, "VI Ref"=w378) -> ("connection info"=w384:T7, "Address Lookup Table Out"=w386:variant)  [unwired: 6 in]
              }
              frame #1 {
                n158 = Tick Count (ms)() -> (millisecond timer value=w388:u32)
              }
            }
            n159 = Bundle By Name(cluster=w364, "DTCs.Timer"=w375, "TCP.Refs"=w362, "Addresses.LUT"=w363) -> (w374:T5)
          }
          frame "Object.Initialize" {
            n160 = call "Initialize Workspace Object.vi"("error in (no error)"=w391, "State"=w393) -> ("error out"=w392:errorcluster)  [unwired: 9 in]
          }
          frame "Object.Configure" {
            n161 = Unbundle By Name(w398) -> ("State"=w400:T4, "State.Notifier"=w403:refnum<user-event>, "NIVS.SysDefRoot"=w404:refnum<k24>, "State.CD Path"=w407:string)
            n162 = call "Select Custom Device.vi"("CD Path"=w407, "NIVS.System Definition Root"=w404) -> ("Cancelled?"=w405:bool, "IP Address"=w408:string, "Custom Device Path Out"=w406:string)  [unwired: 7 in]
            n163 = case shown="False" w405 {
              tunnel: w403 -> [w411 _]
              tunnel: w408 -> [w416 _]
              tunnel: w406 -> [w417 _]
              tunnel: w402 -> [w414 w428]
              tunnel: [w414 w428] -> w401
              tunnel: w400 -> [w415 w427]
              tunnel: [w410 w427] -> w399
              tunnel: w396 -> [w413 w426]
              tunnel: [w412 w426] -> w395
              frame False {
                n164 = flat-sequence {
                  tunnel: w417 -> [w425]
                  tunnel: w416 -> [w424]
                  tunnel: w415 -> [w423]
                  tunnel: w411 -> [w420]
                  tunnel: [w419] -> w410
                  tunnel: [w418] -> _
                  frame #0 {
                    n165 = Bundle By Name(cluster=w423, "CD Path"=w425, "CD IP"=w424) -> (w419:T4)
                    n166 = Bundle By Name(cluster=T17 {"Operation"=enum."SetCustomData", "Data"=variant} ("event data"), "Data"=w419) -> (w421:T17)
                    n167 = Generate User Event(user event=w420, event data cluster=w421) -> (error out=w418:errorcluster)  [unwired: 2 in, 1 out]
                  }
                }
                n168 = Build Array (concatenate)(w413, string[] ["Stream.Disable", "UI.Stream.Disabled", "UI.Log.Enabled", "VS.CheckConnect"]) -> (w412:string[])
              }
              frame True {
              }
            }
            n169 = Bundle By Name(cluster=w398, "State"=w399) -> (w397:T5)
          }
          frame "Object.Connected" {
            n170 = Unbundle By Name(w432) -> ("TCP.Refs"=w430:T7, "State.CD IP"=w435:string, "State.CD Path"=w436:string)
            n171 = call "STM Close Connection.vi"("connection info"=w430) -> ("error out"=w429:errorcluster)  [unwired: 10 in]
            n172 = flat-sequence {
              tunnel: w438 -> [w450]
              tunnel: [w448] -> w437
              tunnel: w436 -> [w440]
              tunnel: w435 -> [w447]
              tunnel: [w445] -> w434
              tunnel: w433 -> [w444]
              tunnel: w432 -> [w442]
              tunnel: [w441] -> w431
              tunnel: w429 -> [_]
              frame #0 {
                n173 = call "UI.Addon.Path.Parse.vi"("Cached Addon Path"=w440) -> ("Addon Name"=w439:string)  [unwired: 6 in, 4 out]
                n174 = call "Open Connection to Target.vi"("error in (no error)"=w444, "IP Address"=w447, "TCP Service"=w439) -> ("error out"=w446:errorcluster, "connection info"=w443:T7)  [unwired: 7 in]
                n175 = Bundle By Name(cluster=w442, "TCP.Refs"=w443) -> (w441:T5)
                n176 = case shown="No Error" w446 {
                  selector: w446 -> [w451 w454]
                  tunnel: [string[] ["Object.Initialize", "UI.Enable"] ("element") string[] ["Object.Initialize", "UI.Disable"] ("element")] -> w449
                  tunnel: [w451 w454] -> w445
                  frame No Error {
                  }
                  frame Error {
                  }
                }
                n177 = Build Array (concatenate)(w450, w449) -> (w448:string[])
              }
            }
          }
          frame "Object.Disconnected" {
            n178 = Unbundle By Name(w460) -> ("TCP.Refs"=w458:T7)
            n179 = Bundle By Name(cluster=w460, "TCP.Refs"=T7 {"connection ID"=refnum, "meta data"=[]}) -> (w459:T5)
            n180 = call "STM Close Connection.vi"("connection info"=w458) -> ()  [unwired: 10 in, 1 out]
          }
          frame "Object.Exit" {
            n181 = Unbundle By Name(w462) -> ("Stream.Qs"=w461:T12)
            n182 = call "Send Host Stream Command Exit.vi"("error in (no error)"=w463, "Q Refs"=w461) -> ("error out"=w464:errorcluster)  [unwired: 9 in]
          }
          frame "VS.CheckConnect" {
            n183 = Unbundle By Name(w471) -> ("UI.Refs.Device"=w478:refnum<vi>, "NIVS.Workspace"=w476:T9, "NIVS.SysDefRoot"=w477:refnum<k24>, "State.CD Path"=w475:string)
            n184 = Current VI's Menubar() -> (w479:refnum<k9>)
            n185 = call "UI.Connection.State.Get.vi"("Menu Ref"=w479, "Name Ref"=w478, "error in (no error)"=w481, "Addon Path in"=w475, "NIVS.System Definition Root in"=w477, "NIVS.Workspace Ref in"=w476) -> ("error out"=w480:errorcluster, "Addon Connected?"=w470:bool, "NIVS.System Definition Root out"=w473:refnum<k24>, "NIVS.Workspace Ref out"=w474:T9, "NIVS.SysDef"=w467:path)  [unwired: 1 in]
            n186 = case shown="True" w470 {
              tunnel: w469 -> [w484 w487]
              tunnel: [w483 w486] -> w468
              frame False {
                n187 = Build Array (concatenate)(w484, string[] ["Object.Disconnected", "Object.Initialize", "UI.Stream.Disabled", "UI.Disable", "Stream.Disable"]) -> (w483:string[])
              }
              frame True {
                n188 = Build Array (concatenate)(w487, string[] ["Object.Connected", "Stream.Filter.Read"]) -> (w486:string[])
              }
            }
            n189 = Bundle By Name(cluster=w471, "NIVS.SysDef"=w467, "NIVS.Workspace"=w474, "NIVS.SysDefRoot"=w473, "Addon.Connected"=w470) -> (w472:T5)
          }
          frame "Stream.Enable" {
            n190 = Unbundle By Name(w494) -> ("Stream.Qs"=w493:T12, "State.CD IP"=w492:string, "State.CD Path"=w491:string, "NIVS.SysDef"=w489:path)
            n191 = call "UI.Addon.Path.Parse.vi"("Cached Addon Path"=w491) -> ("Addon Name"=w490:string)  [unwired: 6 in, 4 out]
            n192 = Strip Path(path=w489) -> (stripped path=w488:path)  [unwired: 1 out]
            n193 = call "Send Host Stream Command Start.vi"("Project Folder"=w488, "error in (no error)"=w495, "Addon"=w490, "Target IP Address"=w492, "Q Refs"=w493) -> ("error out"=w496:errorcluster)  [unwired: 6 in]
          }
          frame "Stream.Filter.Send" {
            n194 = Unbundle By Name(w510) -> ("TCP.Refs"=w509:T7, "State.CD IP"=w512:string, "State.CD Path"=w511:string)
            n195 = local read "Direction Filter"() -> (w500:T3)
            n196 = local read "Type Filter"() -> (w501:T2)
            n197 = local read "Filter IDs"() -> (w499:string)
            n198 = call "Check and Reestablish Connection.vi"("CD Path"=w511, "IP Address"=w512, "connection info"=w509) -> ("error out"=w507:errorcluster, "connection info"=w508:T7)  [unwired: 7 in]
            n199 = call "Convert Filter IDs String to Array.vi"("Filter IDs"=w499) -> ("Filter IDs"=w498:u32[])  [unwired: 10 in]
            n200 = Bundle By Name(cluster=T14 {"ID Filters"=[], "Direction Filter"=enum."Tx/Rx", "Type Filter"=enum."All"} ("IDs"), "ID Filters"=w498, "Direction Filter"=w500, "Type Filter"=w501) -> (w502:T14)
            n201 = call "SetStreamingFilter.vi"("error in (no error)"=w507, "IDs"=w502, "connection info"=w508) -> ("error out"=w505:errorcluster, "connection info"=w506:T7)  [unwired: 7 in]
            n202 = call "Close Connection with CD.vi"("error in (no error)"=w505, "connection info"=w506) -> ("error out"=w504:errorcluster)  [unwired: 9 in]
            n203 = call <vilib>:"Simple Error Handler.vi"("error in (no error)"=w504) -> ()  [unwired: 4 in, 5 out]
          }
          frame "Stream.Filter.Clear" {
            n204 = Unbundle By Name(w517) -> ("TCP.Refs"=w522:T7, "State.CD IP"=w524:string, "State.CD Path"=w523:string)
            n205 = call "Check and Reestablish Connection.vi"("CD Path"=w523, "IP Address"=w524, "connection info"=w522) -> ("error out"=w520:errorcluster, "connection info"=w521:T7)  [unwired: 7 in]
            n206 = call "SetStreamingFilter.vi"("error in (no error)"=w520, "IDs"=T14 {"ID Filters"=[], "Direction Filter"=enum."Tx/Rx", "Type Filter"=enum."All"}, "connection info"=w521) -> ("error out"=w518:errorcluster, "connection info"=w519:T7)  [unwired: 7 in]
            n207 = call "Close Connection with CD.vi"("error in (no error)"=w518, "connection info"=w519) -> ("error out"=w515:errorcluster)  [unwired: 9 in]
            n208 = call <vilib>:"Simple Error Handler.vi"("error in (no error)"=w515) -> ()  [unwired: 4 in, 5 out]
          }
          frame "Stream.Filter.Reset" {
            n209 = Unbundle By Name(w533) -> ("TCP.Refs"=w539:T7, "State.CD IP"=w541:string, "State.CD Path"=w540:string)
            n210 = call "Check and Reestablish Connection.vi"("CD Path"=w540, "IP Address"=w541, "connection info"=w539) -> ("error out"=w537:errorcluster, "connection info"=w538:T7)  [unwired: 7 in]
            n211 = call "ResetStreamingFilter.vi"("error in (no error)"=w537, "connection info"=w538) -> ("error out"=w535:errorcluster, "IDs"=w532:T14, "connection info"=w536:T7)  [unwired: 7 in]
            n212 = Unbundle By Name(w532) -> ("ID Filters"=w530:u32[], "Direction Filter"=w529:T3, "Type Filter"=w528:T2)
            n213 = call "Close Connection with CD.vi"("error in (no error)"=w535, "connection info"=w536) -> ("error out"=w534:errorcluster)  [unwired: 9 in]
            n214 = call <vilib>:"Simple Error Handler.vi"("error in (no error)"=w534) -> ()  [unwired: 4 in, 5 out]
            n215 = call "Convert Filter IDs Array to String.vi"("Filter IDs"=w530) -> ("Filter IDs"=w531:string)  [unwired: 10 in]
            n216 = local write "Host Filter"(FALSE ("Host Filter")) -> ()
            n217 = local write "Filter IDs"(w531) -> ()
            n218 = local write "Direction Filter"(w529) -> ()
            n219 = local write "Type Filter"(w528) -> ()
          }
          frame "Stream.Filter.Read" {
            n220 = Unbundle By Name(w544) -> ("TCP.Refs"=w555:T7, "State.CD IP"=w557:string, "State.CD Path"=w556:string)
            n221 = call "Check and Reestablish Connection.vi"("CD Path"=w556, "IP Address"=w557, "connection info"=w555) -> ("error out"=w553:errorcluster, "connection info"=w554:T7)  [unwired: 7 in]
            n222 = call "ResetStreamingFilter.vi"("error in (no error)"=w553, "connection info"=w554) -> ("error out"=w551:errorcluster, "IDs"=w549:T14, "connection info"=w552:T7)  [unwired: 7 in]
            n223 = Unbundle By Name(w549) -> ("ID Filters"=w547:u32[], "Direction Filter"=w546:T3, "Type Filter"=w545:T2)
            n224 = call "Close Connection with CD.vi"("error in (no error)"=w551, "connection info"=w552) -> ("error out"=w550:errorcluster)  [unwired: 9 in]
            n225 = call <vilib>:"Simple Error Handler.vi"("error in (no error)"=w550) -> ()  [unwired: 4 in, 5 out]
            n226 = call "Convert Filter IDs Array to String.vi"("Filter IDs"=w547) -> ("Filter IDs"=w548:string)  [unwired: 10 in]
            n227 = local write "Filter IDs"(w548) -> ()
            n228 = local write "Direction Filter"(w546) -> ()
            n229 = local write "Type Filter"(w545) -> ()
          }
          frame "Stream.Table.GoUp" {
            n230 = Unbundle By Name(w562) -> ("UI.Refs.Table Control"=w563:refnum<vi>)
            n231 = property class="Tbl (strict)"(reference=w563, error in=w560, "Index Values"=T18 {"Row"=0, "Column"=0}) -> (error out=w561:errorcluster)  [unwired: 1 out]
          }
          frame "Stream.Disable" {
            n232 = Unbundle By Name(w569) -> ("Stream.Qs"=w568:T12)
            n233 = call "Send Host Stream Command Stop.vi"("error in (no error)"=w566, "Q Refs"=w568) -> ("error out"=w567:errorcluster)  [unwired: 9 in]
          }
          frame "Raw.Clear" {
            n234 = Unbundle By Name(w578) -> ("UI.Refs.Identifier"=w576:refnum<vi>, "UI.Refs.Data"=w577:refnum<vi>)
            n235 = property class="Arr (strict)"(reference=w577, error in=w573, "Value"=u8[] []) -> (error out=w575:errorcluster)  [unwired: 1 out]
            n236 = property class="DigNum (strict)"(reference=w576, error in=w575, "Val(Sgnl)"=u32 0 ("Value (Signaling)")) -> (error out=w574:errorcluster)  [unwired: 1 out]
          }
          frame "Raw.Send" {
            n237 = Unbundle By Name(w586) -> ("TCP.Refs"=w590:T7, "State"=w589:T4, "Addresses.LUT"=w588:variant, "Errors.Q"=w584:refnum<queue>, "UI.Refs.ParentVI"=w583:refnum<vi>)
            n238 = call "RAW Event.vi"("connection info"=w590, "State Variables"=w589, "Address Lookup Table"=w588, "Identifier"="Identifier", "Data"="Data", "Error Q"=w584, "VI Ref"=w583) -> ("connection info"=w582:T7, "Address Lookup Table Out"=w581:variant)  [unwired: 7 in]
            n239 = Bundle By Name(cluster=w586, "TCP.Refs"=w582, "Addresses.LUT"=w581) -> (w585:T5)
          }
          frame "Request.Send" {
            n240 = Unbundle By Name(w598) -> ("TCP.Refs"=w603:T7, "State"=w602:T4, "Addresses.LUT"=w601:variant, "Errors.Q"=w600:refnum<queue>, "UI.Refs.ParentVI"=w599:refnum<vi>)
            n241 = call "Request Event.vi"("connection info"=w603, "State Variables"=w602, "Address Lookup Table"=w601, "PGN"="PGN", "DA"="DA", "Error Q"=w600, "VI Ref"=w599) -> ("connection info"=w597:T7, "Response"=→"Response":string, "Address Lookup Table Out"=w596:variant)  [unwired: 6 in]
            n242 = Bundle By Name(cluster=w598, "TCP.Refs"=w597, "Addresses.LUT"=w596) -> (w595:T5)
          }
          frame "UI.Disable" {
            n243 = Unbundle By Name(w608) -> ("Mode.Tool?"=w607:bool, "UI.Refs"=w614:T11)
            n244 = call "Workspace.UI.DisableState.Set.vi"("Mode.Tool?"=w607, "error in (no error)"=w611, "Enable?"=FALSE, "UI.Refs"=w614) -> ("error out"=w610:errorcluster, "UI.Refs out"=w613:T11)  [unwired: 6 in]
            n245 = Bundle By Name(cluster=w608, "UI.Refs"=w613) -> (w609:T5)
          }
          frame "UI.Stream.Enabled" {
            n246 = call "UI.Stream.Enable.vi"("error in (no error)"=w616, "State Variables in"=w618) -> ("error out"=w617:errorcluster)  [unwired: 9 in]
          }
          frame "UI.Log.Enabled" {
            w624 = T16."Disabled and Grayed Out" ("Disabled")
            n247 = Unbundle By Name(w622) -> ("UI.Refs.Type Filter"=w628:refnum<vi>, "UI.Refs.Filter IDs"=w627:refnum<vi>, "UI.Refs.Direction Filter"=w626:refnum<vi>, "UI.Refs.Reset Filter"=w631:refnum<vi>, "UI.Refs.Host Filter"=w633:refnum<vi>)
            n248 = property class="Bool (strict)"(reference=w633, error in=w623, "DisabledEnum"=w624) -> (error out=w632:errorcluster, "Value"=w630:bool)  [unwired: 1 out]
            n249 = Build Array(w628, w627, w626) -> (w625:refnum<vi>[])
            n250 = property class="Bool"(reference=w631, error in=w632, "DisabledEnum"=w624) -> (error out=w629:errorcluster)  [unwired: 1 out]
            n251 = case shown="False" w630 {
              tunnel: w629 -> [w636 w642]
              tunnel: w625 -> [w637 _]
              tunnel: [w635 w642] -> w620
              tunnel: w624 -> [w634 _]
              frame False {
                n252 = for {
                  tunnel: w637 -> [w641] mode=indexing
                  shift-right: [w639] -> w635
                  shift-left: w636 -> [w640]
                  tunnel: w634 -> [w638]
                  n253 = property class="Ctl"(reference=w641, error in=w640, "DisabledEnum"=w638) -> (error out=w639:errorcluster)  [unwired: 1 out]
                }
              }
              frame True {
              }
            }
          }
          frame "UI.Stream.Disabled" {
            n254 = call "UI.Stream.Disable.vi"("error in (no error)"=w644, "State Variables in"=w643) -> ("error out"=w645:errorcluster)  [unwired: 9 in]
          }
          frame "UI.Log.Disabled" {
            w650 = T16."Enabled" ("Disabled")
            n255 = Unbundle By Name(w648) -> ("UI.Refs.Type Filter"=w654:refnum<vi>, "UI.Refs.Filter IDs"=w653:refnum<vi>, "UI.Refs.Direction Filter"=w652:refnum<vi>, "UI.Refs.Reset Filter"=w656:refnum<vi>, "UI.Refs.Host Filter"=w658:refnum<vi>)
            n256 = property class="Bool (strict)"(reference=w658, error in=w649, "DisabledEnum"=w650) -> (error out=w657:errorcluster)  [unwired: 1 out]
            n257 = Build Array(w654, w653, w652) -> (w651:refnum<vi>[])
            n258 = property class="Bool"(reference=w656, error in=w657, "DisabledEnum"=w650) -> (error out=w655:errorcluster)  [unwired: 1 out]
            n259 = for {
              tunnel: w651 -> [w663] mode=indexing
              shift-right: [w661] -> w647
              shift-left: w655 -> [w662]
              tunnel: w650 -> [w660]
              n260 = property class="Ctl"(reference=w663, error in=w662, "DisabledEnum"=w660) -> (error out=w661:errorcluster)  [unwired: 1 out]
            }
          }
          frame "UI.Enable" {
            n261 = Unbundle By Name(w665) -> ("Mode.Tool?"=w664:bool, "UI.Refs"=w671:T11)
            n262 = call "Workspace.UI.DisableState.Set.vi"("Mode.Tool?"=w664, "error in (no error)"=w668, "Enable?"=TRUE, "UI.Refs"=w671) -> ("error out"=w667:errorcluster, "UI.Refs out"=w670:T11)  [unwired: 6 in]
            n263 = Bundle By Name(cluster=w665, "UI.Refs"=w670) -> (w666:T5)
          }
          frame Default {
            n264 = Concatenate Strings(w674, " is not a valid command." ("string")) -> (w673:string)
            n265 = One Button Dialog(message=w673) -> ()  [unwired: 1 in, 1 out]
          }
        }
      }
      frame Error {
        n266 = call <vilib>:"Simple Error Handler.vi"("error in (no error)"=w684) -> ("error out"=w683:errorcluster)  [unwired: 4 in, 4 out]
        n267 = call <vilib>:"Clear Errors.vi"("error in (no error)"=w683) -> ("error out"=w682:errorcluster)  [unwired: 5 in, 1 out]
      }
    }
  }
  n268 = Unbundle By Name(w37) -> ("NIVS.Workspace"=w32:T9, "NIVS.State.Refs"=w33:T10, "State.Notifier"=w35:refnum<user-event>, "LaunchConfig.Ref"=w36:refnum<user-event>, "Events.Refs"=w34:T19, "TCP.Refs"=w31:T7, "Errors.Q"=w28:refnum<queue>)
  n269 = flat-sequence {
    tunnel: w36 -> [w698]
    tunnel: w35 -> [w697]
    tunnel: w34 -> [w696]
    tunnel: w33 -> [w695]
    tunnel: w32 -> [w694]
    tunnel: w31 -> [w688]
    tunnel: w28 -> [w685]
    tunnel: [w693] -> w26
    tunnel: [w692] -> w25
    tunnel: [w691] -> w24
    tunnel: [w690] -> w23
    tunnel: [w689] -> w22
    tunnel: [w687] -> w21
    tunnel: [w686] -> w20
    tunnel: w26 -> [_]
    tunnel: w25 -> [_]
    tunnel: w24 -> [_]
    tunnel: w23 -> [_]
    tunnel: w22 -> [_]
    tunnel: w21 -> [_]
    tunnel: w20 -> [_]
    tunnel: [w699] -> _
    frame #0 {
      n270 = call <vilib>:"NI VeriStand - Close Workspace Manager Reference.vi"("WorkspaceManager"=w694) -> ("error out"=w693:errorcluster)  [unwired: 10 in]
      n271 = call <vilib>:"NI VeriStand - Close Engine State Change Notification.vi"("SystemStateRefs"=w695) -> ("error out"=w692:errorcluster)  [unwired: 10 in]
      n272 = Destroy User Event(user event=w697) -> (error out=w691:errorcluster)  [unwired: 1 in]
      n273 = Destroy User Event(user event=w698) -> (error out=w690:errorcluster)  [unwired: 1 in]
      n274 = Unregister For Events(event registration refnum=w696) -> (error out=w689:errorcluster)  [unwired: 1 in]
      n275 = call "STM Close Connection.vi"("connection info"=w688) -> ("error out"=w687:errorcluster)  [unwired: 10 in]
      n276 = Release Queue(queue=w685) -> (error out=w686:errorcluster)  [unwired: 2 in, 2 out]
    }
    frame #1 {
      n277 = invoke class="VI" method="FP.Close"() -> (error out=w699:errorcluster)  [unwired: 3 in, 2 out]
    }
  }
